vi "lockin - Set REF phase equals zero.vi"(8 "error in (no error)":errorcluster, 11 "LockinDAQ out":refnum<class "LockinDAQ.lvclass">) -> (0 "error out":errorcluster, 3 "LockinDAQ":refnum<class "LockinDAQ.lvclass">)   [LabVIEW 2016, in "LockinDAQ.lvclass"]
uses:
  LockinDAQ.lvclass
  LockinDAQ.lvclass/LockinDAQ.ctl
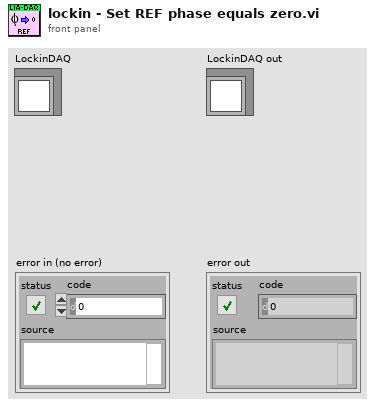
[diagram p1: front panel]
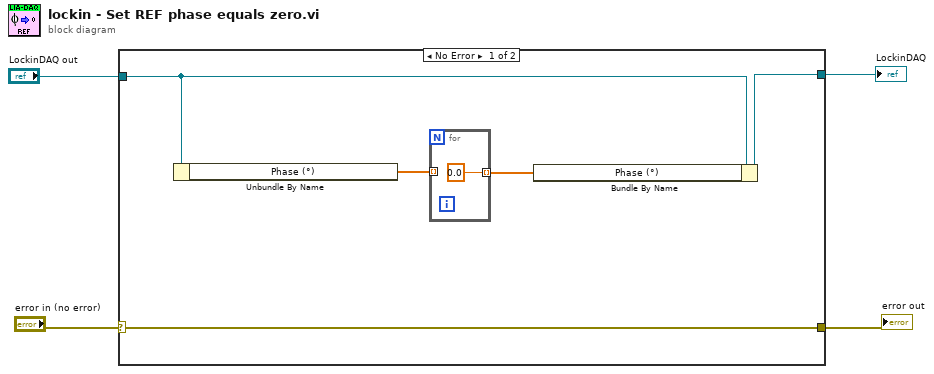
[diagram p0: block diagram]
diagram:
  n1 = case shown="No Error" "error in (no error)" {
    selector: "error in (no error)" -> [w5 w12]
    tunnel: "LockinDAQ out" -> [w9 w11]
    tunnel: [w8 w11] -> w3
    tunnel: [w5 w12] -> w1
    frame No Error {
      n2 = Unbundle By Name(w9) -> ("Phase (°)"=w7:dbl[])
      n3 = for {
        tunnel: [0.0] -> w6 mode=indexing
        tunnel: w7 -> [_] mode=indexing
      }
      n4 = Bundle By Name(cluster=w9, "Phase (°)"=w6) -> (w8:refnum<class "LockinDAQ.lvclass">)
    }
    frame Error {
    }
  }
  "LockinDAQ" <- w3
  "error out" <- w1
